vi "Dokugen Main.vi"(10 "Output Directory Path":path=path "C:/Users/samkristoff/Desktop/output", 11 "Source Directory Path":path=path "C:/Program Files (x86)/National Instruments/LabVIEW 2011/vi.lib/LabVIEW Hacker/LVH-Toolbox/Common/Public") -> ()   [LabVIEW 2014, in "LMH-Toolbox.lvlib" / "LMH-Documentation.lvlib"]
uses:
  <vilib>/MakerHub/Toolbox/Private/Documentation/LMH-Documentation.lvlib
panel:
  in  "Image Base Path":string="lib/exe/fetch.php?media=libraries:lvh_toolbox:vis:"
  in  "GitHub Base Path":string="https://github.com/labviewhacker/LVH-Toolbox/raw/master/LabVIEW/vi.lib/LabVIEW%20Hacker/LVH-Toolbox/Common/Public/"
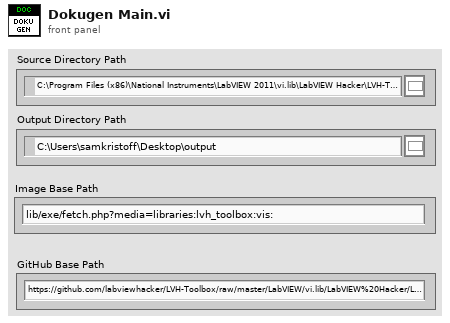
[diagram p1: front panel]
types:
  T1 = typedef "LMH-Toolbox.lvlib/LMH-Documentation.lvlib/Doc Config.ctl" = cluster{"Source Directory":path, "Output Directory":path}
  T2 = typedef "LMH-Toolbox.lvlib/LMH-Documentation.lvlib/VI.ctl" = cluster{"Name":string, "Description":string, "VI Relative Path":string, "Con_Img_Path":string, "BD_Img_Path":string}
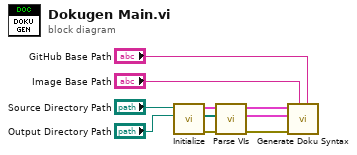
[diagram p0: block diagram]
diagram:
  n1 = call <vilib>:"Initialize.vi"("Output Directory Path"="Output Directory Path", "Source Directory Path"="Source Directory Path") -> ("Error Out"=w10:errorcluster, "All VIs"=w6:path[], "Doc Config"=w9:T1)  [unwired: 7 in]
  n2 = call <vilib>:"Parse VIs.vi"("Error In"=w10, "All VIs"=w6, "Doc Config"=w9) -> ("Error Out"=w3:errorcluster, "VIs"=w5:T2[], "Doc Config"=w4:T1)  [unwired: 6 in]
  n3 = call <vilib>:"Generate Doku Syntax.vi"("GitHub Base Path"="GitHub Base Path", "Image Base Path"="Image Base Path", "Error In"=w3, "VIs"=w5, "Doc Config"=w4) -> ()  [unwired: 6 in, 1 out]
